vi "Framework_Initialize.vi"(8 "error in (no error)":errorcluster, 11 "AB_SourceDistribution in":refnum<class "AB_SourceDistribution.lvclass">) -> (0 "error out":errorcluster, 1 "helpTopics":string[](array[string]), 2 "pageTitles":string[](array[string]), 3 "AB_SourceDistribution out":refnum<class "AB_SourceDistribution.lvclass">, 4 "helpFile":string, 5 "pages":path[](array[path]))   [LabVIEW 2020, in "AB_SourceDistribution.lvclass"]
uses:
  <vilib>/AppBuilder/AB_Classes/SourceDistribution/AB_SourceDistribution.lvclass
panel:
  in  "pageTitles_SDist":string[](array[string])=["Information", "Source Files", "Destinations", "Source File Settings", "Advanced", "Additional Exclusions", "Version Information", "Pre/Post Build Actions", "Preview"]
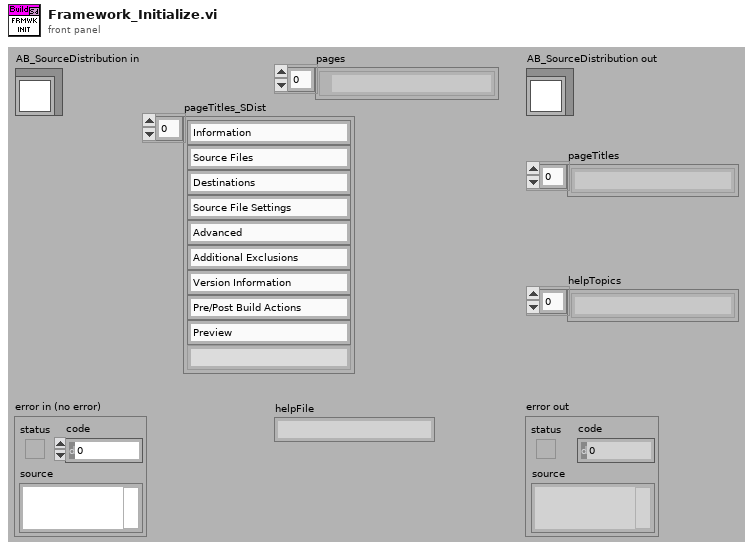
[diagram p1: front panel]
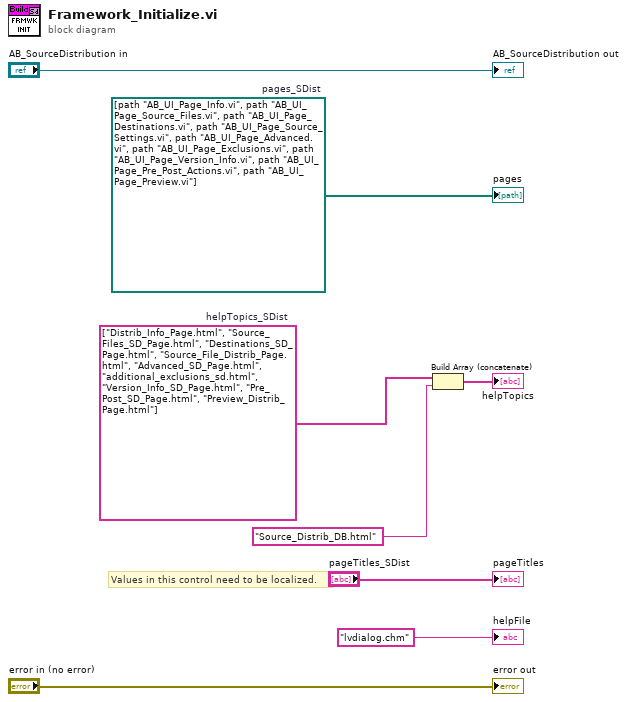
[diagram p0: block diagram]
diagram:
  w3 = string[] ["Distrib_Info_Page.html", "Source_Files_SD_Page.html", "Destinations_SD_Page.html", "Source_File_Distrib_Page.html", "Advanced_SD_Page.html", "additional_exclusions_sd.html", "Version_Info_SD_Page.html", "Pre_Post_SD_Page.html", "Preview_Distrib_Page.html"]  # helpTopics_SDist
  w6 = path[] [path "AB_UI_Page_Info.vi", path "AB_UI_Page_Source_Files.vi", path "AB_UI_Page_Destinations.vi", path "AB_UI_Page_Source_Settings.vi", path "AB_UI_Page_Advanced.vi", path "AB_UI_Page_Exclusions.vi", path "AB_UI_Page_Version_Info.vi", path "AB_UI_Page_Pre_Post_Actions.vi", path "AB_UI_Page_Preview.vi"]  # pages_SDist
  # "Values in this control need to be localized."
  n1 = Build Array (concatenate)(w3, "Source_Distrib_DB.html" ("HTML filename")) -> (→"helpTopics":string[])
  "error out" <- "error in (no error)"
  "AB_SourceDistribution out" <- "AB_SourceDistribution in"
  "pages" <- w6
  "pageTitles" <- "pageTitles_SDist"
  "helpFile" <- "lvdialog.chm" ("CHM or HLP filename (lvdialog.chm)")
